vi "Get Resource ID.vi"(4 "GPIO in":refnum<class "GPIO.lvclass">) -> (7 "Resource ID":string)   [LabVIEW 2024, in "CTI.lvlib" / "GPIO.lvclass"]
uses:
  GPIO.lvclass
  GPIO.lvclass/GPIO.ctl
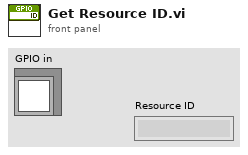
[diagram p1: front panel]
types:
  T1 = typedef "CTI.lvlib/GPIO Number.ctl" = i8
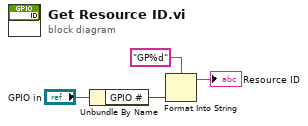
[diagram p0: block diagram]
diagram:
  n1 = Unbundle By Name("GPIO in") -> ("GPIO #"=w3:T1)
  n2 = Format Into String(format string="GP%d", w3) -> (resulting string=→"Resource ID":string)  [unwired: 2 in, 1 out]
